vi "Update Progress.vi"(4 "Total Operations (1)":i32=1, 6 "Current Operation (0)":i32, 8 "error in":errorcluster, 9 "Current Iteration":i32, 10 "Total Interations":i32, 11 "Operation":string) -> (0 "error out":errorcluster)   [LabVIEW 2013, in "LVTM.lvlib"]
uses:
  LVTM.lvlib
  Controls_LVTM/Status.ctl
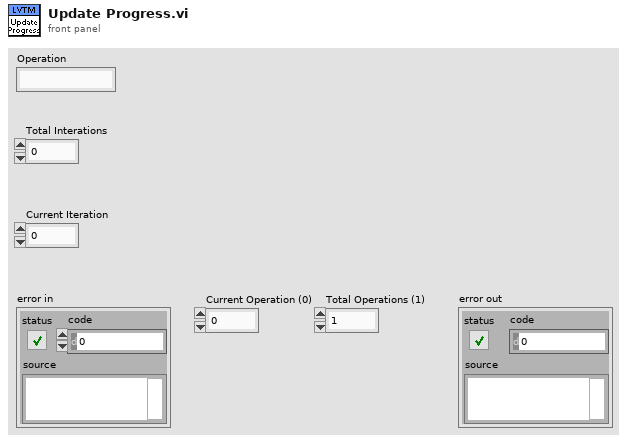
[diagram p1: front panel]
types:
  T1 = typedef "LVTM.lvlib/Status.ctl" = cluster{"Operation":string, "Total Interations":i32, "Current Iteration":i32, "Total Operations":i32, "Current Operation":i32}
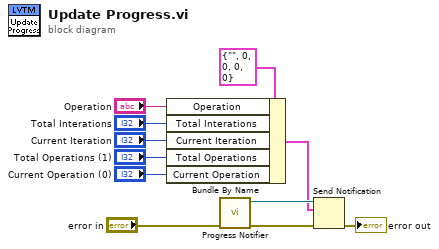
[diagram p0: block diagram]
diagram:
  n1 = Bundle By Name(cluster=T1 {"Operation"="", "Total Interations"=0, "Current Iteration"=0, "Total Operations"=0, "Current Operation"=0} ("notification"), "Operation"="Operation", "Total Interations"="Total Interations", "Current Iteration"="Current Iteration", "Total Operations"="Total Operations (1)", "Current Operation"="Current Operation (0)") -> (w6:T1)
  n2 = call "Progress Notifier.vi"("error in"="error in") -> ("error out"=w9:errorcluster, "notifier out"=w8:refnum<notifier>)  [unwired: 9 in]
  n3 = Send Notification(notification=w6, notifier=w8, error in (no error)=w9) -> (error out=→"error out":errorcluster)  [unwired: 1 out]
